vi "Global LQIdentity Registry.vi"(8 "Error In":errorcluster, 9 "Registry Action":T1=enum."Deregister LQIdentity", 10 "LQIdentity Info In":refnum<class "LQIdentity.lvclass">) -> (0 "Error Out":errorcluster, 2 "LQIdentity Info Out":refnum<class "LQIdentity.lvclass">)   [LabVIEW 2013, in "Template.lvlib" / "LQCoreEngine.lvclass"]
uses:
  LQCoreEngine.lvclass
  LQIdentity Registry Action.ctl
  LQIdentity/LQIdentity.lvclass
  LQIdentity/LQIdentity.lvclass/LQIdentity.ctl
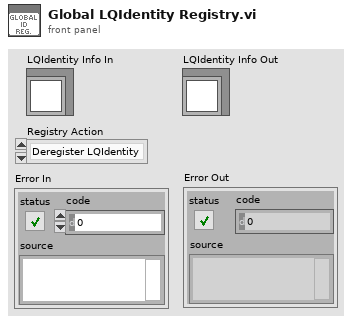
[diagram p1: front panel]
types:
  T1 = typedef "Template.lvlib/LQCoreEngine.lvclass/LQIdentity Registry Action.ctl" = enum16{"Init", "Register LQIdentity", "Get LQIdentity Info", "Deregister LQIdentity"}
  T2 = enum16{"big-endian, network order", "native, host order", "little-endian"}
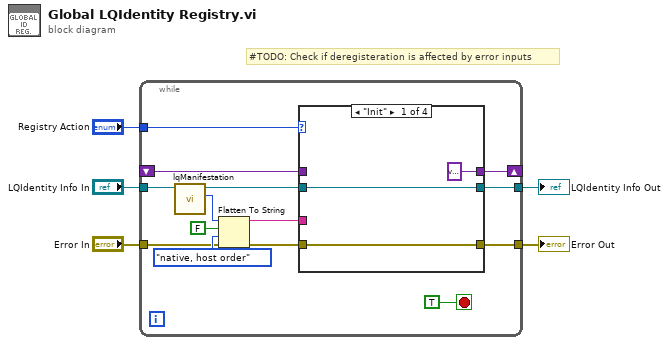
[diagram p0: block diagram]
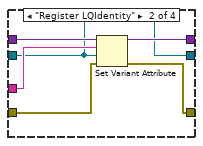
[diagram p2: hidden frame]
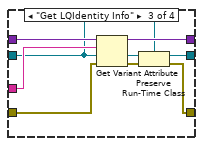
[diagram p3: hidden frame]
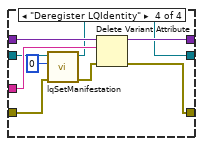
[diagram p4: hidden frame]
diagram:
  # "#TODO: Check if deregisteration is affected by error inputs"
  n1 = while {
    tunnel: "Registry Action" -> [w19]
    shift-right: [w17] -> _
    shift-left: _ -> [w16]
    tunnel: "LQIdentity Info In" -> [w15]
    tunnel: [w9] -> w3
    tunnel: "Error In" -> [w8]
    tunnel: [w6] -> w1
    stop <- TRUE stop-if-true
    n2 = call "lqManifestation.vi"("LQIdentity in"=w15) -> ("Manifestation"=w12:u64, "LQIdentity out"=w10:refnum<class "LQIdentity.lvclass">)  [unwired: 9 in]
    n3 = Flatten To String(anything=w12, prepend array or string size? (T)=FALSE, byte order (0:big-endian, network order)=T2."native, host order", error in (no error)=w8) -> (data string=w11:string, error out=w7:errorcluster)  [unwired: 1 out]
    n4 = case shown="\"Init\"" w19 {
      tunnel: [variant ("Dup. Signal Map") w27 w36 w45] -> w17
      tunnel: w16 -> [_ w28 w37 w46]
      tunnel: w11 -> [_ w26 w35 w44]
      tunnel: w10 -> [w20 w25 w29 w42]
      tunnel: [w20 w25 w32 w38] -> w9
      tunnel: w7 -> [w21 w24 w34 w41]
      tunnel: [w21 w23 w30 w43] -> w6
      frame "Init" {
      }
      frame "Register LQIdentity" {
        n5 = Set Variant Attribute(Variant=w28, name=w26, value=w25, error in=w24) -> (Variant out=w27:variant, error out=w23:errorcluster)  [unwired: 1 out]
      }
      frame "Get LQIdentity Info" {
        n6 = Get Variant Attribute(Variant=w37, name=w35, default value (empty Variant)=w29, error in=w34) -> (duplicate Variant=w36:variant, value=w33:refnum<class "LQIdentity.lvclass">, error out=w31:errorcluster)  [unwired: 1 out]
        n7 = Preserve Run-Time Class(object in=w33, error in=w31, 2:w29) -> (object out=w32:refnum<class "LQIdentity.lvclass">, error out=w30:errorcluster)
      }
      frame "Deregister LQIdentity" {
        n8 = call "lqSetManifestation.vi"("Error In"=w41, "Manifestation"=u64 0, "LQIdentity in"=w42) -> ("Error Out"=w40:errorcluster, "LQIdentity out"=w38:refnum<class "LQIdentity.lvclass">)  [unwired: 7 in]
        n9 = Delete Variant Attribute(4:w40, 6:w44, 7:w46) -> (0:w43:errorcluster, 3:w45:variant)  [unwired: 1 out]
      }
    }
  }
  "LQIdentity Info Out" <- w3
  "Error Out" <- w1
